vi "XYZ-For-IRC.vi"() -> ()   [LabVIEW 2019]
panel:
  out "離開越質範圍":bool
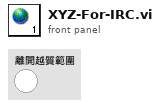
[diagram p1: front panel]
diagram:
